vi "final_control_mk7_022825.vi"() -> ()   [LabVIEW 2023]
doc: "Simplified example program for initializing the COM port, determining the data frame of up to 26 Alicats, acquiring the data of the same number of Alicats, displaying the data of the one with the selected unit ID, and writing a setpoint to the same selected unit ID.\n\nThis is a slightly more feature rich version of the Alicat Simplified Driver Example, and contains an example of a method for interfacing with up to 26 Alicats on a single COM port by means of for loops with shift registers to handle sequential commands to each included Alicat. This also contains a method to write a setpoint to the same selected unit.\n\nIf coding for multiple Alicats on a single COM port without the use of for loops with shift registers, ensure that each Alicat command is executed sequentially. Alicat's RS-232/485 does not work if multiple devices are responding simultaneously."
uses:
  <vilib>/Platform/TimedLoop/XDataNode/timing_clust.ctl
  <vilib>/Platform/TimedLoop/XDataNode/nitl_modes.ctl
  <vilib>/Platform/TimedLoop/XDataNode/wakeup.ctl
  <vilib>/DAQmx/write.llb/DAQmx Write (Analog 1D DBL NChan 1Samp).vi
  <vilib>/DAQmx/read.llb/DAQmx Read (Analog 1D DBL 1Chan NSamp).vi
  <extravilib>/ChannelInstances/Tag-bool/Read With Abort.vi
  <extravilib>/ChannelInstances/Tag-bool/Write With Abort.vi
  <vilib>/Utility/file.llb/Write Delimited Spreadsheet (string).vi
  <extravilib>/ChannelInstances/Tag-bool/Instantiate.vi
  <vilib>/Utility/file.llb/Read Delimited Spreadsheet (DBL).vi
  <extravilib>/ChannelInstances/Tag-bool/EndpointRead.vi
  <vilib>/DAQmx/miscellaneous.llb/DAQmx Fill In Error Info.vi
  <extravilib>/ChannelInstances/Tag-bool/Endpoint.vi
  <vilib>/platform/TimedLoop/XDataNode/XDataNode.xnode
  <vilib>/Platform/TimedLoop/XDataNode/XDNodeRunTimeDep.lvlib
  <extravilib>/ChannelInstances/Tag-bool.lvlib
panel:
  in  "Tab Control":enum32{"Page 1", "Page 2"}(tab)
  in  "COM Port Settings":T1={"Baud Rate"=enum."19200", "VISA Sesssion In"="MassFlowControllers"}
  out "Range Exceeded":bool
  out "Error Present":bool
  out "Error Text":string
  out "Elapsed Time [ms]\n(all units)":dbl caption="Elapsed Time (s)"
  in  "Minimum time between \nreadings [ms] (all units)":u32
  in  "Device ID's \nto Include:":T2={"A"=TRUE, "B"=TRUE, "C"=TRUE, "D"=TRUE, "E"=TRUE, "F"=TRUE, "G"=FALSE, "H"=FALSE, "I"=FALSE, "J"=FALSE, "K"=FALSE, "L"=FALSE, "M"=FALSE, "N"=FALSE, "O"=FALSE, "P"=FALSE, "Q"=FALSE, "R"=FALSE, "S"=FALSE, "T"=FALSE, "U"=FALSE, "V"=FALSE, "W"=FALSE, "X"=FALSE, "Y"=FALSE, "Z"=FALSE}
  out "Active Device":u16(ring) items=["A", "B", "C", "D", "E", "F"]
  out "Meas. Data (for active device)":T3
  in  "Write File":path
  in  "Hold Time\n[min]":dbl=17.0 min=17.0
  out "Global Start Time":i64
  out "N":i32
  out "Iteration Duration":i64
  in  "Read File":path
  in  "End Program":bool
  in  "Start From:":i32
  out "len_SP":i32
  out "Setpoints":dbl[][](array[numeric])=[[4.2, 3.3], [69.0, 4.2]]
  out "Z":dbl[](array[numeric])
  out "ASP":dbl
  out "BSP":dbl
  out "CSP":dbl
  out "DSP":dbl
  out "ESP":dbl
  out "FSP":dbl
  out "N_i_read":dbl
  out "N_read":i32
  out "read count":dbl=2.0
  out "T_SCh":string[](array[string])
  out "Iter_#":string
  out "V_D":string
  out "V_H":string
  out "Iter_Duration":string
  out "all rows":dbl[][](array[numeric])
  # "Totalizer Timer"
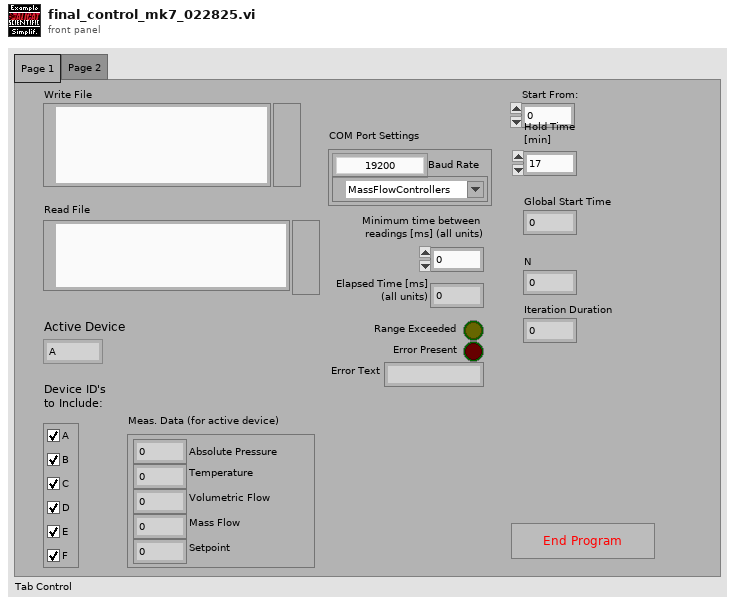
[diagram p1: front panel]
types:
  T1 = cluster{"Baud Rate":enum8{"2400", "9600", "19200", "38400", "57600", "115200", "Unknown"}, "VISA Sesssion In":refnum<visa-resource-name>}
  T2 = cluster{"A":bool, "B":bool, "C":bool, "D":bool, "E":bool, "F":bool, "G":bool, "H":bool, "I":bool, "J":bool, "K":bool, "L":bool, "M":bool, "N":bool, "O":bool, "P":bool, "Q":bool, "R":bool, "S":bool, "T":bool, "U":bool, "V":bool, "W":bool, "X":bool, "Y":bool, "Z":bool}
  T3 = cluster{"Absolute Pressure":dbl, "Gauge/Diff. Pressure":dbl, "Barometric Pressure":dbl, "Temperature":dbl, "Volumetric Flow":dbl, "Mass Flow":dbl, "Setpoint":dbl, "Valve Drive":dbl, "Totalizer":dbl, "[hr]":dbl, "[min]":dbl, "[sec]":dbl, "Totalizer Average Flow":dbl, "Totalizer Peak Flow":dbl, "Gas selected":string}
  T4 = cluster{"Unit ID":string, "Baud Rate":enum8{"2400", "9600", "19200", "38400", "57600", "115200", "Unknown"}, "VISA Sesssion In":refnum<visa-resource-name>}
  T5 = typedef "XDNodeRunTimeDep.lvlib/timing_clust.ctl" = cluster{"Expected End [f-1]":u64, "Actual End [f-1]":u64, "Finished Late? [f-1]":bool, "Expected End [i-1]":u64, "Actual End [i-1]":u64, "Finished Late? [i-1]":bool, "Expected Start [i]":u64, "Actual Start [i]":u64, "Expected Start [f]":u64, "Actual Start [f]":u64, "Source Name":string, "Structure Name":string, "Period":i64, "Deadline":i64, "Offset":i64, "Start":i64, "Priority":i32, "Timeout":i32, "Mode":T6, "Wakeup Reason":T7, "Error":errorcluster, "Source Type":string, "Secondary Source Type":string, "Global End Time":u64, "Global Start Time":u64, "Frame Duration":u64, "Iteration Duration":u64, "Assigned CPU":i32, "I/O Scan Engine Mode":u32}
  T6 = typedef "XDNodeRunTimeDep.lvlib/nitl_modes.ctl" = enum32{"No Change", "Process missed periods, maintain original phase", "Discard missed periods, maintain original phase", "Process missed periods, ignore original phase", "Discard missed periods, ignore original phase"}
  T7 = typedef "XDNodeRunTimeDep.lvlib/wakeup.ctl" = enum32{"Normal", "Aborted", "Asynchronous wakeup", "Timing source error", "Timed loop error", "Timeout"}
  T8 = typedef "Tag-bool.lvlib/))Channel.ctl" = refnum<queue>
  T9 = enum8{"2400", "9600", "19200", "38400", "57600", "115200", "Unknown"}
  T10 = cluster{"Absolute Pressure":bool, "Gauge/Diff. Pressure":bool, "Barometric Pressure":bool, "Temperature":bool, "Volumetric":bool, "Mass":bool, "Setpoint":bool, "Valve Drive":bool, "Totalizer":bool, "Totalizer Timer":bool, "Totalizer Average Flow":bool, "Totalizer Peak Flow":bool, "Gas Selected":bool, "Tot. Timer Format":u16}
  T11 = cluster{"Controller Full Scale":dbl, "Controller Select":u16, "Control Range":enum16{"Normal", "Inverted", "Bidirectional", "Unknown"}}
  T12 = cluster{"Controller Full Scale":dbl, "Controller Select":u16, "Control Range":enum16{"Normal", "Inverted", "Bidirectional", "Unknown"}}[]
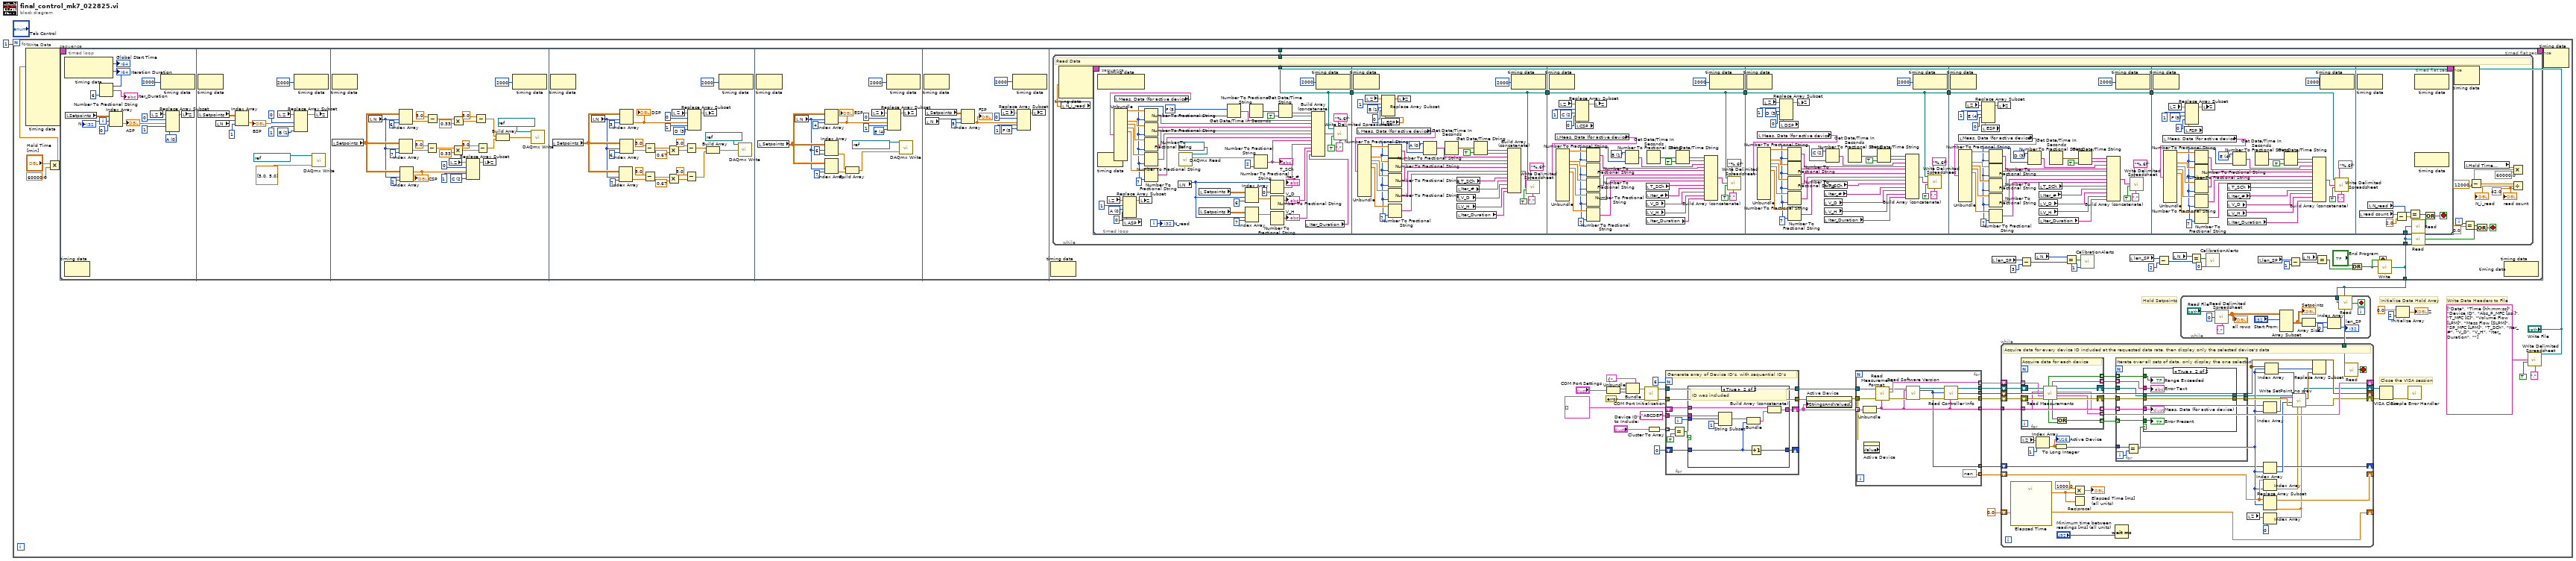
[diagram p0: block diagram]
diagram:
  n1 = for {
    N: 1 -> [_]
    # "Write Data Headers to File"
    # "Hold Setpoints"
    # "Initialize Data Hold Array"
    # "Close the VISA session"
    n2 = Multiply(x="Hold Time\n[min]", y=60000.0) -> (x*y=w2:dbl)
    n3 = node-c288(w2) -> (w43:T5)  [unwired: 9 in]
    n4 = timed-loop "Write Data" {
      timing: w43 -> [_]
      timing-out: [_] -> w42
      tunnel: [w56] -> w9
      tunnel: "Write File" -> [w55]
      i -> [w70]
      stop <- w210 stop-if-true
      n5 = timed-sequence {
        timing: _ -> [_]
        timing-out: _ -> [_]
        tunnel: [w58] -> w56
        tunnel: w55 -> [w57]
        n6 = timed-flat-sequence {
          tunnel: [w205] -> w58
          tunnel: w57 -> [w206]
          frame #0 {
            w64 = u16 0 items=["A", "B", "C", "D", "E", "F"]
            n7 = node-c288() -> (→"Global Start Time":i64, w63:i64)  [unwired: 1 in]
            "Iteration Duration" <- w63
            n8 = local read "Setpoints"() -> (w72:dbl[][])
            n9 = Number To Fractional String(number=w63, precision (6)=i16 6) -> (F-format string=→"Iter_Duration":string)  [unwired: 2 in]
            n10 = Index Array(array=w72, index (row)=w70, index (col)=0 ("index (row)")) -> (element=w69:dbl)
            "ASP" <- w69
            n11 = local read "Z"() -> (w67:dbl[])
            n12 = node-c288(i64 2000 ("Start")) -> ()  [unwired: 1 out]
            n13 = Replace Array Subset(array=w67, new element #1=w69, index #1=0 ("index"), new element #2=w64, index #2=1 ("index")) -> (w68:dbl[])
            n14 = local write "Z"(w68) -> ()
            "N" <- w70
          }
          frame #1 {
            w81 = u16 1 items=["A", "B", "C", "D", "E", "F"]
            n15 = node-c288() -> ()  [unwired: 1 in, 1 out]
            n16 = local read "Setpoints"() -> (w89:dbl[][])
            n17 = local read "N"() -> (w82:i32)
            n18 = Index Array(array=w89, index (row)=w82, index (col)=1 ("index (row)")) -> (element=w86:dbl)
            "BSP" <- w86
            n19 = local read "Z"() -> (w84:dbl[])
            n20 = Replace Array Subset(array=w84, new element #1=w86, index #1=0 ("index"), new element #2=w81, index #2=1 ("index")) -> (w85:dbl[])
            n21 = node-c288(i64 2000 ("Start")) -> ()  [unwired: 1 out]
            n22 = call-poly <vilib>:"DAQmx Write.vi"("task/channels in"=refnum<k21> "Valve_cont", "data"=dbl[] [5.0, 5.0]) -> ()  [unwired: 11 in, 3 out]
            n23 = local write "Z"(w85) -> ()
          }
          frame #2 {
            w96 = u16 2 items=["A", "B", "C", "D", "E", "F"]
            n24 = node-c288() -> ()  [unwired: 1 in, 1 out]
            n25 = local read "Setpoints"() -> (w108:dbl[][])
            n26 = local read "N"() -> (w107:i32)
            n27 = Index Array(array=w108, index (row)=w107, index (col)=6 ("disabled index (col)")) -> (element=w98:dbl)
            n28 = Index Array(array=w108, index (row)=w107, index (col)=7 ("disabled index (col)")) -> (element=w106:dbl)
            n29 = Index Array(array=w108, index (row)=w107, index (col)=2 ("index (row)")) -> (element=w120:dbl)
            "CSP" <- w120
            n30 = Subtract(x=5.0, y=w106) -> (x-y=w115:dbl)
            n31 = Subtract(x=5.0, y=w98) -> (x-y=w102:dbl)
            n32 = local read "Z"() -> (w118:dbl[])
            n33 = Multiply(x=w115, y=0.33) -> (x*y=w113:dbl)
            n34 = Multiply(x=w102, y=0.33) -> (x*y=w100:dbl)
            n35 = Replace Array Subset(array=w118, new element #1=w120, index #1=0 ("index"), new element #2=w96, index #2=1 ("index")) -> (w119:dbl[])
            n36 = Subtract(x=5.0, y=w100) -> (x-y=w97:dbl)
            n37 = Subtract(x=5.0, y=w113) -> (x-y=w110:dbl)
            n38 = local write "Z"(w119) -> ()
            n39 = Build Array(w97, w110) -> (w109:dbl[])
            n40 = node-c288(i64 2000 ("Start")) -> ()  [unwired: 1 out]
            n41 = call-poly <vilib>:"DAQmx Write.vi"("task/channels in"=refnum<k21> "Valve_cont", "data"=w109) -> ()  [unwired: 11 in, 3 out]
          }
          frame #3 {
            w147 = u16 3 items=["A", "B", "C", "D", "E", "F"]
            n42 = node-c288() -> ()  [unwired: 1 in, 1 out]
            n43 = local read "Setpoints"() -> (w136:dbl[][])
            n44 = local read "N"() -> (w135:i32)
            n45 = Index Array(array=w136, index (row)=w135, index (col)=7 ("disabled index (col)")) -> (element=w128:dbl)
            n46 = Index Array(array=w136, index (row)=w135, index (col)=3 ("index (row)")) -> (element=w151:dbl)
            "DSP" <- w151
            n47 = Index Array(array=w136, index (row)=w135, index (col)=6 ("disabled index (col)")) -> (element=w134:dbl)
            n48 = Subtract(x=5.0, y=w134) -> (x-y=w144:dbl)
            n49 = Subtract(x=5.0, y=w128) -> (x-y=w132:dbl)
            n50 = Multiply(x=w144, y=0.67) -> (x*y=w142:dbl)
            n51 = Multiply(x=w132, y=0.67) -> (x*y=w130:dbl)
            n52 = local read "Z"() -> (w149:dbl[])
            n53 = Subtract(x=5.0, y=w142) -> (x-y=w138:dbl)
            n54 = Subtract(x=5.0, y=w130) -> (x-y=w127:dbl)
            n55 = Replace Array Subset(array=w149, new element #1=w151, index #1=0 ("index"), new element #2=w147, index #2=1 ("index")) -> (w150:dbl[])
            n56 = local write "Z"(w150) -> ()
            n57 = Build Array(w138, w127) -> (w137:dbl[])
            n58 = node-c288(i64 2000 ("Start")) -> ()  [unwired: 1 out]
            n59 = call-poly <vilib>:"DAQmx Write.vi"("task/channels in"=refnum<k21> "Valve_cont", "data"=w137) -> ()  [unwired: 11 in, 3 out]
          }
          frame #4 {
            w168 = u16 4 items=["A", "B", "C", "D", "E", "F"]
            n60 = node-c288() -> ()  [unwired: 1 in, 1 out]
            n61 = local read "Setpoints"() -> (w163:dbl[][])
            n62 = local read "N"() -> (w162:i32)
            n63 = Index Array(array=w163, index (row)=w162, index (col)=4 ("index (row)")) -> (element=w172:dbl)
            "ESP" <- w172
            n64 = Index Array(array=w163, index (row)=w162, index (col)=6 ("disabled index (col)")) -> (element=w165:dbl)
            n65 = Index Array(array=w163, index (row)=w162, index (col)=7 ("disabled index (col)")) -> (element=w164:dbl)
            n66 = Build Array(w165, w164) -> (w161:dbl[])
            n67 = local read "Z"() -> (w170:dbl[])
            n68 = node-c288(i64 2000 ("Start")) -> ()  [unwired: 1 out]
            n69 = Replace Array Subset(array=w170, new element #1=w172, index #1=0 ("index"), new element #2=w168, index #2=1 ("index")) -> (w171:dbl[])
            n70 = call-poly <vilib>:"DAQmx Write.vi"("task/channels in"=refnum<k21> "Valve_cont", "data"=w161) -> ()  [unwired: 11 in, 3 out]
            n71 = local write "Z"(w171) -> ()
          }
          frame #5 {
            w182 = u16 5 items=["A", "B", "C", "D", "E", "F"]
            n72 = node-c288() -> ()  [unwired: 1 in, 1 out]
            n73 = local read "Setpoints"() -> (w185:dbl[][])
            n74 = local read "N"() -> (w180:i32)
            n75 = Index Array(array=w185, index (row)=w180, index (col)=5 ("index (row)")) -> (element=w181:dbl)
            "FSP" <- w181
            n76 = local read "Z"() -> (w184:dbl[])
            n77 = node-c288(i64 2000 ("Start")) -> ()  [unwired: 1 out]
            n78 = Replace Array Subset(array=w184, new element #1=w181, index #1=0 ("index"), new element #2=w182, index #2=1 ("index")) -> (w183:dbl[])
            n79 = local write "Z"(w183) -> ()
          }
          frame #6 {
            n80 = node-c288() -> ()  [unwired: 1 in, 1 out]
            n81 = local read "len_SP"() -> (w194:i32)
            n82 = Subtract(x=w194, y=3) -> (x-y=w196:i32)
            n83 = local read "N"() -> (w195:i32)
            n84 = Equal?(x=w195, y=w196) -> (x = y?=w197:bool)
            n85 = call "CalibrationAlerts.vi"("Alert Type (0)"=1, "Trigger"=w197) -> ()  [unwired: 10 in]
            n86 = local read "len_SP"() -> (w200:i32)
            n87 = Subtract(x=w200, y=2) -> (x-y=w199:i32)
            n88 = local read "N"() -> (w204:i32)
            n89 = Equal?(x=w204, y=w199) -> (x = y?=w202:bool)
            n90 = call "CalibrationAlerts.vi"("Alert Type (0)"=0, "Trigger"=w202) -> ()  [unwired: 10 in]
            n91 = local read "len_SP"() -> (w209:i32)
            n92 = Subtract(x=w209, y=1) -> (x-y=w212:i32)
            n93 = local read "N"() -> (w208:i32)
            n94 = Equal?(x=w208, y=w212) -> (x = y?=w211:bool)
            n95 = Or(x="End Program", y=w211) -> (x .or. y?=w210:bool)
            n96 = call <extravilib>:"Write.vi"("element"=w210) -> ("channel"=w205:T8)  [unwired: 1 out]
            n97 = while {
              tunnel: w206 -> [w228]
              tunnel: w205 -> [w215]
              i -> [w214]
              stop <- w224 stop-if-true
              w218 = 42.0 ("y")
              # "Read Data"
              n98 = local read "N_i_read"() -> (w223:dbl)
              n99 = node-c288(w223) -> (w230:T5)  [unwired: 2 in]
              n100 = timed-loop {
                timing: w230 -> [_]
                timing-out: [_] -> w229
                tunnel: w228 -> [w231]
                tunnel: w215 -> [w232]
                i -> [w286]
                stop <- w487 stop-if-true
                n101 = timed-sequence {
                  timing: _ -> [_]
                  timing-out: _ -> [_]
                  tunnel: w232 -> [w234]
                  tunnel: w231 -> [w233]
                  n102 = timed-flat-sequence {
                    tunnel: [w245] -> w239
                    tunnel: w233 -> [w245]
                    tunnel: w239 -> [w311]
                    tunnel: [w311] -> w238
                    tunnel: w238 -> [w341]
                    tunnel: [w341] -> w237
                    tunnel: w237 -> [w376]
                    tunnel: [w376] -> w236
                    tunnel: w236 -> [w441]
                    tunnel: [w441] -> w235
                    tunnel: w235 -> [w453]
                    tunnel: w234 -> [w486]
                    frame #0 {
                      w262 = u16 5 items=["A", "B", "C", "D", "E", "F"]
                      w265 = u16 0 items=["A", "B", "C", "D", "E", "F"]
                      w257 = i16 7 ("precision (6)")
                      n103 = node-c288() -> ()  [unwired: 1 in, 1 out]
                      n104 = local read "Z"() -> (w249:dbl[])
                      n105 = local read "Meas. Data (for active device)"() -> (w246:T3)
                      n106 = Unbundle(w246) -> ("Absolute Pressure"=w273:dbl, "Temperature"=w260:dbl, "Volumetric Flow"=w269:dbl, "Mass Flow"=w259:dbl, "Setpoint"=w258:dbl)  [unwired: 10 out]
                      n107 = local read "ASP"() -> (w247:dbl)
                      n108 = Replace Array Subset(array=w249, new element #1=w265, index #1=1 ("index"), new element #2=w247, index #2=0 ("index")) -> (w248:dbl[])
                      n109 = local write "Z"(w248) -> ()
                      n110 = Number To Fractional String(number=w273, precision (6)=w257) -> (F-format string=w254:string)  [unwired: 2 in]
                      n111 = Number To Fractional String(number=w260, precision (6)=w257) -> (F-format string=w252:string)  [unwired: 2 in]
                      n112 = Number To Fractional String(number=w269, precision (6)=w257) -> (F-format string=w253:string)  [unwired: 2 in]
                      n113 = Number To Fractional String(number=w259, precision (6)=w257) -> (F-format string=w251:string)  [unwired: 2 in]
                      n114 = Number To Fractional String(number=w258, precision (6)=w257) -> (F-format string=w250:string)  [unwired: 2 in]
                      n115 = local read "N"() -> (w280:i32)
                      n116 = call-poly <vilib>:"DAQmx Read.vi"("task/channels in"=refnum<k21> "T_SCh") -> ("data"=w276:dbl[])  [unwired: 12 in, 2 out]
                      n117 = local read "Setpoints"() -> (w283:dbl[][])
                      n118 = local read "Setpoints"() -> (w279:dbl[][])
                      n119 = Number To Fractional String(number=w262, precision (6)=w257) -> (F-format string=w255:string)  [unwired: 2 in]
                      n120 = Index Array(array=w283, index (row)=w280, index (col)=6 ("disabled index (col)")) -> (element=w282:dbl)
                      n121 = Index Array(array=w279, index (row)=w280, index (col)=7 ("disabled index (col)")) -> (element=w281:dbl)
                      n122 = Get Date/Time In Seconds() -> (seconds since 1Jan1904=w268:timestamp)
                      n123 = Number To Fractional String(number=w276, precision (6)=i16 2) -> (F-format string=w240:string[])  [unwired: 2 in]
                      "T_SCh" <- w240
                      n124 = Number To Fractional String(number=w280, precision (6)=i16 0) -> (F-format string=w241:string)  [unwired: 2 in]
                      "Iter_#" <- w241
                      n125 = Number To Fractional String(number=w282) -> (F-format string=w242:string)  [unwired: 3 in]
                      "V_D" <- w242
                      n126 = Number To Fractional String(number=w281) -> (F-format string=w243:string)  [unwired: 3 in]
                      "V_H" <- w243
                      n127 = Get Date/Time String(seconds (now)=w268, want seconds? (F)=TRUE) -> (date string=w267:string, time string=w256:string)  [unwired: 1 in]
                      n128 = local read "Iter_Duration"() -> (w244:string)
                      n129 = Build Array (concatenate)(w267, w256, w255, w254, w252, w253, w251, w250, w240, w241, w242, w243, w244) -> (w270:string[])
                      n130 = node-c288(i64 2000 ("Start")) -> ()  [unwired: 1 out]
                      n131 = call-poly <vilib>:"Write Delimited Spreadsheet.vi"("file path (dialog if empty)"=w245, "format (%s)"="%.6f" ("format (%.3f)"), "1D data"=w270, "append to file? (new file:F)"=TRUE, "delimiter (\\t)"="," ("delimiter (\\t)")) -> ()  [unwired: 9 in, 2 out]
                      "N_read" <- w286
                    }
                    frame #1 {
                      w308 = u16 0 items=["A", "B", "C", "D", "E", "F"]
                      w317 = u16 1 items=["A", "B", "C", "D", "E", "F"]
                      w303 = i16 7 ("precision (6)")
                      n132 = node-c288() -> ()  [unwired: 1 in, 1 out]
                      n133 = local read "Meas. Data (for active device)"() -> (w315:T3)
                      n134 = Unbundle(w315) -> ("Absolute Pressure"=w325:dbl, "Temperature"=w306:dbl, "Volumetric Flow"=w321:dbl, "Mass Flow"=w305:dbl, "Setpoint"=w304:dbl)  [unwired: 10 out]
                      n135 = local read "Z"() -> (w314:dbl[])
                      n136 = local read "BSP"() -> (w309:dbl)
                      n137 = Replace Array Subset(array=w314, new element #1=w317, index #1=1 ("index"), new element #2=w309, index #2=0 ("index")) -> (w313:dbl[])
                      n138 = Number To Fractional String(number=w325, precision (6)=w303) -> (F-format string=w300:string)  [unwired: 2 in]
                      n139 = Number To Fractional String(number=w306, precision (6)=w303) -> (F-format string=w298:string)  [unwired: 2 in]
                      n140 = Number To Fractional String(number=w321, precision (6)=w303) -> (F-format string=w299:string)  [unwired: 2 in]
                      n141 = Number To Fractional String(number=w305, precision (6)=w303) -> (F-format string=w297:string)  [unwired: 2 in]
                      n142 = Number To Fractional String(number=w304, precision (6)=w303) -> (F-format string=w296:string)  [unwired: 2 in]
                      n143 = local write "Z"(w313) -> ()
                      n144 = Number To Fractional String(number=w308, precision (6)=w303) -> (F-format string=w301:string)  [unwired: 2 in]
                      n145 = Get Date/Time In Seconds() -> (seconds since 1Jan1904=w320:timestamp)
                      n146 = local read "T_SCh"() -> (w295:string[])
                      n147 = local read "Iter_#"() -> (w294:string)
                      n148 = local read "V_D"() -> (w293:string)
                      n149 = local read "V_H"() -> (w292:string)
                      n150 = local read "Iter_Duration"() -> (w291:string)
                      n151 = Get Date/Time String(seconds (now)=w320, want seconds? (F)=TRUE) -> (date string=w319:string, time string=w302:string)  [unwired: 1 in]
                      n152 = Build Array (concatenate)(w319, w302, w301, w300, w298, w299, w297, w296, w295, w294, w293, w292, w291) -> (w322:string[])
                      n153 = node-c288(i64 2000 ("Start")) -> ()  [unwired: 1 out]
                      n154 = call-poly <vilib>:"Write Delimited Spreadsheet.vi"("file path (dialog if empty)"=w311, "format (%s)"="%.6f" ("format (%.3f)"), "1D data"=w322, "append to file? (new file:F)"=TRUE, "delimiter (\\t)"="," ("delimiter (\\t)")) -> ()  [unwired: 9 in, 2 out]
                    }
                    frame #2 {
                      w349 = u16 1 items=["A", "B", "C", "D", "E", "F"]
                      w346 = i16 7 ("precision (6)")
                      w363 = u16 2 items=["A", "B", "C", "D", "E", "F"]
                      n155 = node-c288() -> ()  [unwired: 1 in, 1 out]
                      n156 = local read "Meas. Data (for active device)"() -> (w352:T3)
                      n157 = Unbundle(w352) -> ("Absolute Pressure"=w357:dbl, "Temperature"=w355:dbl, "Volumetric Flow"=w356:dbl, "Mass Flow"=w354:dbl, "Setpoint"=w353:dbl)  [unwired: 10 out]
                      n158 = local read "Z"() -> (w362:dbl[])
                      n159 = local read "CSP"() -> (w358:dbl)
                      n160 = Replace Array Subset(array=w362, new element #1=w363, index #1=1 ("index"), new element #2=w358, index #2=0 ("index")) -> (w361:dbl[])
                      n161 = Number To Fractional String(number=w357, precision (6)=w346) -> (F-format string=w334:string)  [unwired: 2 in]
                      n162 = Number To Fractional String(number=w355, precision (6)=w346) -> (F-format string=w333:string)  [unwired: 2 in]
                      n163 = Number To Fractional String(number=w356, precision (6)=w346) -> (F-format string=w332:string)  [unwired: 2 in]
                      n164 = Number To Fractional String(number=w354, precision (6)=w346) -> (F-format string=w331:string)  [unwired: 2 in]
                      n165 = Number To Fractional String(number=w353, precision (6)=w346) -> (F-format string=w330:string)  [unwired: 2 in]
                      n166 = local write "Z"(w361) -> ()
                      n167 = Number To Fractional String(number=w349, precision (6)=w346) -> (F-format string=w335:string)  [unwired: 2 in]
                      n168 = local read "T_SCh"() -> (w340:string[])
                      n169 = local read "Iter_#"() -> (w339:string)
                      n170 = local read "V_D"() -> (w338:string)
                      n171 = local read "V_H"() -> (w337:string)
                      n172 = local read "Iter_Duration"() -> (w336:string)
                      n173 = Get Date/Time In Seconds() -> (seconds since 1Jan1904=w351:timestamp)
                      n174 = Get Date/Time String(seconds (now)=w351, want seconds? (F)=TRUE) -> (date string=w350:string, time string=w347:string)  [unwired: 1 in]
                      n175 = Build Array (concatenate)(w350, w347, w335, w334, w333, w332, w331, w330, w340, w339, w338, w337, w336) -> (w342:string[])
                      n176 = node-c288(i64 2000 ("Start")) -> ()  [unwired: 1 out]
                      n177 = call-poly <vilib>:"Write Delimited Spreadsheet.vi"("file path (dialog if empty)"=w341, "format (%s)"="%.6f" ("format (%.3f)"), "1D data"=w342, "append to file? (new file:F)"=TRUE, "delimiter (\\t)"="," ("delimiter (\\t)")) -> ()  [unwired: 9 in, 2 out]
                    }
                    frame #3 {
                      w370 = u16 3 items=["A", "B", "C", "D", "E", "F"]
                      w395 = u16 2 items=["A", "B", "C", "D", "E", "F"]
                      w392 = i16 7 ("precision (6)")
                      n178 = node-c288() -> ()  [unwired: 1 in, 1 out]
                      n179 = local read "Meas. Data (for active device)"() -> (w375:T3)
                      n180 = Unbundle(w375) -> ("Absolute Pressure"=w402:dbl, "Temperature"=w400:dbl, "Volumetric Flow"=w401:dbl, "Mass Flow"=w399:dbl, "Setpoint"=w398:dbl)  [unwired: 10 out]
                      n181 = local read "Z"() -> (w373:dbl[])
                      n182 = local read "DSP"() -> (w374:dbl)
                      n183 = Replace Array Subset(array=w373, new element #1=w370, index #1=1 ("index"), new element #2=w374, index #2=0 ("index")) -> (w372:dbl[])
                      n184 = Number To Fractional String(number=w402, precision (6)=w392) -> (F-format string=w386:string)  [unwired: 2 in]
                      n185 = Number To Fractional String(number=w400, precision (6)=w392) -> (F-format string=w385:string)  [unwired: 2 in]
                      n186 = Number To Fractional String(number=w401, precision (6)=w392) -> (F-format string=w384:string)  [unwired: 2 in]
                      n187 = Number To Fractional String(number=w399, precision (6)=w392) -> (F-format string=w383:string)  [unwired: 2 in]
                      n188 = Number To Fractional String(number=w398, precision (6)=w392) -> (F-format string=w382:string)  [unwired: 2 in]
                      n189 = local write "Z"(w372) -> ()
                      n190 = local read "T_SCh"() -> (w377:string[])
                      n191 = local read "Iter_#"() -> (w378:string)
                      n192 = local read "V_D"() -> (w379:string)
                      n193 = local read "V_H"() -> (w380:string)
                      n194 = local read "Iter_Duration"() -> (w381:string)
                      n195 = Number To Fractional String(number=w395, precision (6)=w392) -> (F-format string=w387:string)  [unwired: 2 in]
                      n196 = Get Date/Time In Seconds() -> (seconds since 1Jan1904=w397:timestamp)
                      n197 = Get Date/Time String(seconds (now)=w397, want seconds? (F)=TRUE) -> (date string=w396:string, time string=w393:string)  [unwired: 1 in]
                      n198 = Build Array (concatenate)(w396, w393, w387, w386, w385, w384, w383, w382, w377, w378, w379, w380, w381) -> (w388:string[])
                      n199 = node-c288(i64 2000 ("Start")) -> ()  [unwired: 1 out]
                      n200 = call-poly <vilib>:"Write Delimited Spreadsheet.vi"("file path (dialog if empty)"=w376, "format (%s)"="%.6f" ("format (%.3f)"), "1D data"=w388, "append to file? (new file:F)"=TRUE, "delimiter (\\t)"="," ("delimiter (\\t)")) -> ()  [unwired: 9 in, 2 out]
                    }
                    frame #4 {
                      w412 = u16 4 items=["A", "B", "C", "D", "E", "F"]
                      w433 = u16 3 items=["A", "B", "C", "D", "E", "F"]
                      w430 = i16 7 ("precision (6)")
                      n201 = node-c288() -> ()  [unwired: 1 in, 1 out]
                      n202 = local read "Meas. Data (for active device)"() -> (w414:T3)
                      n203 = Unbundle(w414) -> ("Absolute Pressure"=w440:dbl, "Temperature"=w438:dbl, "Volumetric Flow"=w439:dbl, "Mass Flow"=w437:dbl, "Setpoint"=w436:dbl)  [unwired: 10 out]
                      n204 = local read "Z"() -> (w409:dbl[])
                      n205 = local read "ESP"() -> (w410:dbl)
                      n206 = Replace Array Subset(array=w409, new element #1=w412, index #1=1 ("index"), new element #2=w410, index #2=0 ("index")) -> (w408:dbl[])
                      n207 = Number To Fractional String(number=w440, precision (6)=w430) -> (F-format string=w424:string)  [unwired: 2 in]
                      n208 = Number To Fractional String(number=w438, precision (6)=w430) -> (F-format string=w423:string)  [unwired: 2 in]
                      n209 = Number To Fractional String(number=w439, precision (6)=w430) -> (F-format string=w422:string)  [unwired: 2 in]
                      n210 = Number To Fractional String(number=w437, precision (6)=w430) -> (F-format string=w421:string)  [unwired: 2 in]
                      n211 = Number To Fractional String(number=w436, precision (6)=w430) -> (F-format string=w420:string)  [unwired: 2 in]
                      n212 = local write "Z"(w408) -> ()
                      n213 = Number To Fractional String(number=w433, precision (6)=w430) -> (F-format string=w425:string)  [unwired: 2 in]
                      n214 = local read "T_SCh"() -> (w419:string[])
                      n215 = local read "Iter_#"() -> (w415:string)
                      n216 = local read "V_D"() -> (w416:string)
                      n217 = local read "V_H"() -> (w417:string)
                      n218 = local read "Iter_Duration"() -> (w418:string)
                      n219 = Get Date/Time In Seconds() -> (seconds since 1Jan1904=w435:timestamp)
                      n220 = Get Date/Time String(seconds (now)=w435, want seconds? (F)=TRUE) -> (date string=w434:string, time string=w431:string)  [unwired: 1 in]
                      n221 = Build Array (concatenate)(w434, w431, w425, w424, w423, w422, w421, w420, w419, w415, w416, w417, w418) -> (w426:string[])
                      n222 = node-c288(i64 2000 ("Start")) -> ()  [unwired: 1 out]
                      n223 = call-poly <vilib>:"Write Delimited Spreadsheet.vi"("format (%s)"="%.6f" ("format (%.3f)"), "1D data"=w426, "append to file? (new file:F)"=TRUE, "delimiter (\\t)"="," ("delimiter (\\t)")) -> ()  [unwired: 10 in, 2 out]
                    }
                    frame #5 {
                      w451 = u16 5 items=["A", "B", "C", "D", "E", "F"]
                      w473 = u16 4 items=["A", "B", "C", "D", "E", "F"]
                      w470 = i16 7 ("precision (6)")
                      n224 = node-c288() -> ()  [unwired: 1 in, 1 out]
                      n225 = local read "Meas. Data (for active device)"() -> (w454:T3)
                      n226 = Unbundle(w454) -> ("Absolute Pressure"=w480:dbl, "Temperature"=w478:dbl, "Volumetric Flow"=w479:dbl, "Mass Flow"=w477:dbl, "Setpoint"=w476:dbl)  [unwired: 10 out]
                      n227 = local read "Z"() -> (w447:dbl[])
                      n228 = local read "FSP"() -> (w449:dbl)
                      n229 = Replace Array Subset(array=w447, new element #1=w451, index #1=1 ("index"), new element #2=w449, index #2=0 ("index")) -> (w448:dbl[])
                      n230 = Number To Fractional String(number=w480, precision (6)=w470) -> (F-format string=w464:string)  [unwired: 2 in]
                      n231 = Number To Fractional String(number=w478, precision (6)=w470) -> (F-format string=w463:string)  [unwired: 2 in]
                      n232 = Number To Fractional String(number=w479, precision (6)=w470) -> (F-format string=w462:string)  [unwired: 2 in]
                      n233 = Number To Fractional String(number=w477, precision (6)=w470) -> (F-format string=w461:string)  [unwired: 2 in]
                      n234 = Number To Fractional String(number=w476, precision (6)=w470) -> (F-format string=w460:string)  [unwired: 2 in]
                      n235 = local write "Z"(w448) -> ()
                      n236 = local read "T_SCh"() -> (w455:string[])
                      n237 = local read "Iter_#"() -> (w456:string)
                      n238 = local read "V_D"() -> (w457:string)
                      n239 = local read "V_H"() -> (w458:string)
                      n240 = local read "Iter_Duration"() -> (w459:string)
                      n241 = Number To Fractional String(number=w473, precision (6)=w470) -> (F-format string=w465:string)  [unwired: 2 in]
                      n242 = Get Date/Time In Seconds() -> (seconds since 1Jan1904=w475:timestamp)
                      n243 = Get Date/Time String(seconds (now)=w475, want seconds? (F)=TRUE) -> (date string=w474:string, time string=w471:string)  [unwired: 1 in]
                      n244 = Build Array (concatenate)(w474, w471, w465, w464, w463, w462, w461, w460, w455, w456, w457, w458, w459) -> (w466:string[])
                      n245 = node-c288(i64 2000 ("Start")) -> ()  [unwired: 1 out]
                      n246 = call-poly <vilib>:"Write Delimited Spreadsheet.vi"("file path (dialog if empty)"=w453, "format (%s)"="%.6f" ("format (%.3f)"), "1D data"=w466, "append to file? (new file:F)"=TRUE, "delimiter (\\t)"="," ("delimiter (\\t)")) -> ()  [unwired: 9 in, 2 out]
                    }
                    frame #6 {
                      n247 = node-c288() -> ()  [unwired: 1 in, 1 out]
                      n248 = local read "read count"() -> (w493:dbl)
                      n249 = local read "N_read"() -> (w491:i32)
                      n250 = Subtract(x=w493, y=2.0) -> (x-y=w492:dbl)
                      n251 = Equal?(x=w491, y=w492) -> (x = y?=w490:bool)
                      n252 = call <extravilib>:"Read.vi"("channel"=w486) -> ("element"=w489:bool)  [unwired: 1 in, 1 out]
                      n253 = node-c288() -> ()  [unwired: 1 in, 1 out]
                      n254 = Or(x=w490, y=w489) -> (x .or. y?=w487:bool)
                    }
                  }
                }
                n255 = node-c288() -> ()  [unwired: 1 in, 1 out]
                n256 = node-c288() -> ()  [unwired: 1 in, 1 out]
              }
              n257 = call <extravilib>:"Read.vi"("channel"=w215) -> ("element"=w225:bool)  [unwired: 1 in, 1 out]
              n258 = node-c288(w229) -> ()  [unwired: 1 out]
              n259 = Equal?(x=w214, y=0.0) -> (x = y?=w226:bool)
              n260 = local read "Hold Time\n[min]"() -> (w221:dbl)
              n261 = Or(x=w226, y=w225) -> (x .or. y?=w224:bool)
              n262 = Multiply(x=w221, y=60000.0) -> (x*y=w220:dbl)
              n263 = Subtract(x=w220, y=12000.0) -> (x-y=w217:dbl)
              n264 = Divide(x=w217, y=w218) -> (x/y=→"N_i_read":dbl)
              "read count" <- w218
            }
            n265 = node-c288() -> ()  [unwired: 1 in, 1 out]
          }
        }
      }
      n266 = node-c288() -> ()  [unwired: 1 in, 1 out]
      n267 = node-c288() -> ()  [unwired: 1 in, 1 out]
    }
    n268 = Unbundle("COM Port Settings") -> ("Baud Rate"=w34:T9, "VISA Sesssion In"=w33:refnum<visa-resource-name>)
    n269 = Bundle(cluster=T4 {"Unit ID"="A", "Baud Rate"=enum."19200", "VISA Sesssion In"="COM1"} ("Communication Settings"), "Baud Rate"=w34, "VISA Sesssion In"=w33) -> (w32:T4)  [unwired: 1 in]
    n270 = call "COM Port Initialization.vi"("error in (no error)"=errorcluster {"status"=FALSE, "code"=0, "source"=""}, "Communication Settings"=w32) -> ("error out"=w25:errorcluster, "VISA Session Out"=w24:refnum<visa-resource-name>)  [unwired: 8 in]
    n271 = Cluster To Array(cluster="Device ID's \nto Include:") -> (array=w28:bool[])
    n272 = for {
      N: 6 -> [_]
      tunnel: "ABCDEF" -> [w534]
      tunnel: w28 -> [w527] mode=indexing
      shift-right: [w526] -> _
      shift-left: u16 0 ("length (rest)") -> [w532]
      shift-right: [w531] -> w22
      shift-left: cluster{string, u16}[] [] -> [w530]
      tunnel: w25 -> [w525]
      tunnel: w24 -> [w524]
      tunnel: [w525] -> w15
      tunnel: [w524] -> w23
      i -> [w533]
      # "Generate array of Device ID's, with sequential ID's"
      n273 = Equal?(x=w527, y=TRUE) -> (x = y?=w529:bool)
      n274 = case shown="True" w529 {
        tunnel: w534 -> [_ w545]
        tunnel: w533 -> [_ w544]
        tunnel: w532 -> [w535 w537]
        tunnel: [w536 w540] -> w531
        tunnel: w530 -> [w536 w538]
        tunnel: [w535 w541] -> w526
        frame False {
          # "ID was not included"
        }
        frame True {
          # "ID was included"
          n275 = String Subset(string=w545, offset (0)=w544, length (rest)=1 ("length (rest)")) -> (substring=w542:string)
          n276 = Bundle(w542, "length (rest)"=w537) -> (w539:cluster{string, "length (rest)":u16})  [unwired: 1 in]
          n277 = Increment(x=w537) -> (x+1=w541:u16)
          n278 = Build Array (concatenate)(w538, w539) -> (w540:cluster{string, "length (rest)":u16}[])
        }
      }
    }
    n279 = property on="Active Device" class="Ring (strict)"(error in=w15, "StringsAndValues[]"=w22) -> (error out=w14:errorcluster)  [unwired: 1 in, 1 out]
    n280 = for {
      tunnel: w23 -> [w522]
      tunnel: [w519] -> w19
      tunnel: w14 -> [w523]
      tunnel: [w518] -> w18
      tunnel: w22 -> [w520] mode=indexing
      tunnel: [w521] -> w21 mode=indexing
      tunnel: [w511] -> w20 mode=indexing
      tunnel: [w517] -> w17 mode=indexing
      tunnel: [nan ("Setpoint")] -> w16 mode=indexing
      tunnel: [w510] -> w13 mode=indexing
      # "Get measurement formats, unit ID's and the controller info"
      n281 = Unbundle(w520) -> (w511:string)  [unwired: 1 out]
      n282 = property on="Active Device" class="Ring (strict)" props=["Value"]() -> ()  [unwired: 2 in, 3 out]
      n283 = call "Read Measurement Format.vi"("Unit ID (A)"=w511, "error in"=w523, "VISA Session In"=w522) -> ("error out"=w514:errorcluster, "Data Frame Format"=w521:T10, "VISA Session Out"=w515:refnum<visa-resource-name>)  [unwired: 6 in]
      n284 = call "Read Software Version.vi"("Unit ID (A)"=w511, "error in"=w514, "VISA Session In"=w515) -> ("error out"=w513:errorcluster, "Software Version"=w510:u8, "VISA Session Out"=w512:refnum<visa-resource-name>)  [unwired: 6 in]
      n285 = call "Read Controller Info.vi"("Unit ID (A)"=w511, "error in"=w513, "Software Version"=w510, "VISA Session In"=w512) -> ("error out"=w518:errorcluster, "Controller Info out"=w517:T11, "VISA Session Out"=w519:refnum<visa-resource-name>)  [unwired: 4 in, 1 out]
    }
    n286 = while {
      shift-right: [w582] -> _
      shift-left: 0.0 ("Set Start Time (s)") -> [w585]
      shift-right: [w568] -> w37
      shift-left: w18 -> [w584]
      shift-right: [w549] -> w38
      shift-left: w19 -> [w583]
      tunnel: w20 -> [w547]
      shift-right: [w570] -> _
      shift-left: w21 -> [w577]
      shift-right: [w567] -> _
      shift-left: w17 -> [w565]
      shift-right: [w563] -> _
      shift-left: w16 -> [w562]
      shift-right: [w558] -> _
      shift-left: w13 -> [w558]
      tunnel: w9 -> [w556]
      stop <- w557 stop-if-true
      # "Acquire data for every device ID included at the requested data rate, then display only the selected device's data"
      n287 = call "Elapsed Time"("Set Start Time (s)"=w585) -> ("Get Start Time (s)"=w582:dbl, "Elapsed Time (s)"=w579:dbl)  [unwired: 11 in, 6 out]
      n288 = for {
        shift-right: [w614] -> w576
        shift-left: w584 -> [w617]
        shift-right: [w615] -> w575
        shift-left: w583 -> [w616]
        tunnel: w577 -> [w611] mode=indexing
        tunnel: w547 -> [w610] mode=indexing
        tunnel: [w609] -> w574 mode=indexing
        tunnel: [w608] -> w573 mode=indexing
        tunnel: [w607] -> w572 mode=indexing
        tunnel: [w606] -> w571 mode=indexing
        tunnel: [w605] -> w570 mode=indexing
        # "Acquire data for each device"
        n289 = call "Read Measurements.vi"("error in"=w617, "Data Frame Format In"=w611, "Unit ID (A)"=w610, "VISA Session In"=w616) -> ("error out"=w614:errorcluster, "Data Frame Format Out"=w605:T10, "Data Cluster"=w608:T3, "VISA Session Out"=w615:refnum<visa-resource-name>, "Unknown Dataframe Info"=w613:bool, "Error/Overrange/Unknown String"=w607:string, "Error Present"=w612:bool, "Range Exceeded"=w606:bool)
        n290 = Or(x=w613, y=w612) -> (x .or. y?=w609:bool)
      }
      n291 = local read "Z"() -> (w553:dbl[])
      n292 = Index Array(array=w553, index=1 ("index (row)")) -> (element=w551:dbl)
      "Active Device" <- w551
      n293 = To Long Integer(number=w551) -> (32bit integer=w560:i32)
      n294 = Multiply(x=1000.0 ("y"), y=w579) -> (x*y=→"Elapsed Time [ms]\n(all units)":dbl)
      n295 = Reciprocal(x=w579) -> ()  [unwired: 1 out]
      n296 = Wait (ms)(milliseconds to wait="Minimum time between \nreadings [ms] (all units)") -> ()  [unwired: 1 out]
      n297 = for {
        tunnel: w576 -> [w588]
        tunnel: [w587] -> w569
        tunnel: w575 -> [w589]
        tunnel: [w586] -> w548
        tunnel: w574 -> [w594] mode=indexing
        tunnel: w560 -> [w596]
        tunnel: w573 -> [w593] mode=indexing
        tunnel: w572 -> [w592] mode=indexing
        tunnel: w571 -> [w591] mode=indexing
        i -> [w595]
        # "Iterate over all sets of data, only display the one selected"
        n298 = Equal?(x=w596, y=w595) -> (x = y?=w590:bool)
        n299 = case shown="True" w590 {
          tunnel: w594 -> [_ w604]
          tunnel: w593 -> [_ w599]
          tunnel: w592 -> [_ w603]
          tunnel: w591 -> [_ w602]
          tunnel: w589 -> [w598 w600]
          tunnel: w588 -> [w597 w601]
          tunnel: [w597 w601] -> w587
          tunnel: [w598 w600] -> w586
          frame False {
            # "Do nothing"
          }
          frame True {
            # "Display data"
            "Range Exceeded" <- w602
            "Error Present" <- w604
            "Error Text" <- w603
            "Meas. Data (for active device)" <- w599
          }
        }
      }
      n300 = local read "Z"() -> (w555:dbl[])
      n301 = Index Array(array=w558, index=w560) -> (element=w559:u8)
      n302 = Index Array(array=w562, index=w560) -> (element=w550:dbl)
      n303 = Index Array(array=w555, index=0) -> (element=w546:dbl)
      n304 = Replace Array Subset(array=w562, new element=w546, index=w560) -> (w563:dbl[])
      n305 = Index Array(array=w547, index=w560) -> (element=w561:string)
      n306 = Index Array(array=w565, index=w560) -> (element=w564:T11)
      n307 = call "Write SetPoint_no prev.vi"("Setpoint"=w546, "Previous Setpoint"=w550, "Unit ID (A)"=w561, "error in"=w569, "Software Version"=w559, "Controller Info out"=w564, "VISA Session In"=w548) -> ("error out"=w568:errorcluster, "Controller Info out"=w566:T11, "VISA Session Out"=w549:refnum<visa-resource-name>)  [unwired: 1 in, 1 out]
      n308 = Replace Array Subset(array=w565, new element=w566, index=w560) -> (w567:T12)
      n309 = call <extravilib>:"Read.vi"("channel"=w556) -> ("element"=w557:bool)  [unwired: 1 in, 1 out]
    }
    n310 = while "Hold Setpoints" {
      tunnel: w9 -> [w50]
      stop <- w51 stop-if-true
      n311 = call-poly <vilib>:"Read Delimited Spreadsheet.vi"("file path (dialog if empty)"="Read File", "start of read offset (chars.:0)"=0, "delimiter (\\t)"="," ("delimiter (\\t)")) -> ("all rows"=w46:dbl[][])  [unwired: 7 in, 5 out]
      "all rows" <- w46
      n312 = Array Subset(array=w46, index (row)="Start From:") -> (w44:dbl[][])  [unwired: 3 in]
      "Setpoints" <- w44
      n313 = Array Size(array=w44) -> (size(s)=w53:i32[])
      n314 = Index Array(array=w53, index=0) -> (element=→"len_SP":i32)
      n315 = call <extravilib>:"Read.vi"("channel"=w50) -> ("element"=w51:bool)  [unwired: 1 in, 1 out]
    }
    n316 = VISA Close(VISA resource name=w38, error in (no error)=w37) -> (error out=w39:errorcluster)
    n317 = Initialize Array(0.0 ("element"), 2 ("dimension size")) -> (→"Z":dbl[])
    n318 = call <vilib>:"Simple Error Handler.vi"("error in (no error)"=w39) -> ()  [unwired: 4 in, 5 out]
    n319 = call-poly <vilib>:"Write Delimited Spreadsheet.vi"("file path (dialog if empty)"="Write File", "1D data"=string[] ["Date", "Time [hh:mm:ss]", "Device ID", "Abs_P_MFC [psi]", "T_MFC [C]", "Volume Flow [LPM]", "Mass Flow [SLPM]", "SP_MFC [LPM]", "T_SCh", "Iter_#", "V_D", "V_H", "Iter_Duration", ""], "append to file? (new file:F)"=TRUE, "delimiter (\\t)"="," ("delimiter (\\t)")) -> ()  [unwired: 10 in, 2 out]
    n320 = node-c288(w42) -> ()  [unwired: 1 out]
  }
